vi "Tosca-Plot DI Data.vi"(0 "state in":T2, 5 "Data":cluster{dbl[][], "DI":bool[][]}, 11 "error in (no error)":errorcluster, 12 "Digital":refnum<vi>, 13 "Controls":T1) -> (4 "state out":T2, 15 "error out":errorcluster)   [LabVIEW 2020]
uses:
  Typedefs/Tosca-AI Plot State.ctl
  Typedefs/Tosca-AI Live Controls.ctl
  epl-vi-lib/Utility VIs/Array Manipulation VIs/Array-Dimensions (2D).vi
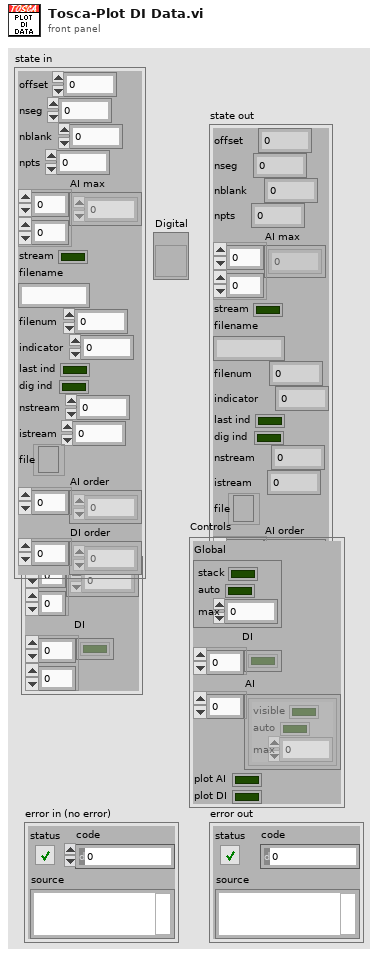
[diagram p1: front panel]
types:
  T1 = typedef "Tosca-AI Live Controls.ctl" = cluster{"Global":cluster{"stack":bool, "auto":bool, "max":dbl}, "DI":bool[], "AI":cluster{"visible":bool, "auto":bool, "max":dbl}[], "plot AI":bool, "plot DI":bool}
  T2 = typedef "Tosca-AI Plot State.ctl" = cluster{"offset":i32, "nseg":i32, "nblank":i32, "npts":i32, "AI max":dbl[][], "stream":bool, "filename":string, "filenum":i32, "indicator":i32, "last ind":bool, "dig ind":bool, "nstream":i32, "istream":i32, "file":refnum<file>, "AI order":i32[], "DI order":i32[]}
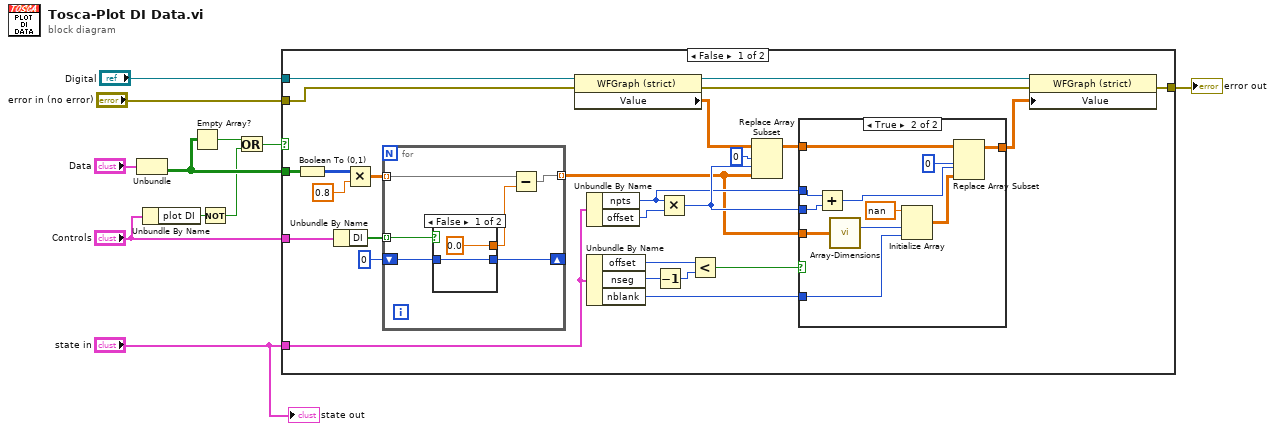
[diagram p0: block diagram]
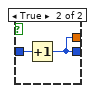
[diagram p2: hidden frame]
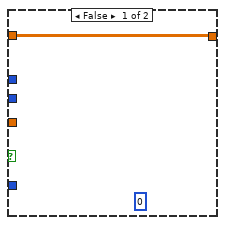
[diagram p3: hidden frame]
diagram:
  n1 = Unbundle("Data") -> ("DI"=w6:bool[][])  [unwired: 1 out]
  n2 = Unbundle By Name("Controls") -> ("plot DI"=w2:bool)
  n3 = Empty Array?(array=w6) -> (empty?=w4:bool)
  n4 = Not(x=w2) -> (.not. x?=w1:bool)
  n5 = Or(x=w4, y=w1) -> (x .or. y?=w3:bool)
  n6 = case shown="False" w3 {
    tunnel: "Digital" -> [w37 _]
    tunnel: "error in (no error)" -> [w36 w60]
    tunnel: "state in" -> [w21 _]
    tunnel: "Controls" -> [w19 _]
    tunnel: [w17 w60] -> w8
    tunnel: w6 -> [w14 _]
    frame False {
      n7 = Boolean To (0,1)(Boolean=w14) -> (0, 1=w12:i16[][])
      n8 = Unbundle By Name(w19) -> ("DI"=w20:bool[])
      n9 = Multiply(x=w12, y=0.8) -> (x*y=w15:dbl[][])
      n10 = for {
        tunnel: w15 -> [w42] mode=indexing
        tunnel: [w43] -> w22 mode=indexing
        tunnel: w20 -> [w38] mode=indexing
        shift-right: [w40] -> _
        shift-left: 0 -> [w41]
        n11 = case shown="False" w38 {
          tunnel: w41 -> [w45 w47]
          tunnel: [w45 w46] -> w40
          tunnel: [0.0 w46] -> w39
          frame False {
          }
          frame True {
            n12 = Increment(x=w47) -> (x+1=w46:i32)
          }
        }
        n13 = Subtract(x=w42, y=w39) -> (x-y=w43:dbl[])
      }
      n14 = property class="WFGraph (strict)"(reference=w37, error in=w36) -> (reference out=w34:refnum<vi>, error out=w33:errorcluster, "Value"=w13:dbl[][])
      n15 = Unbundle By Name(w21) -> ("npts"=w24:i32, "offset"=w32:i32)
      n16 = Unbundle By Name(w21) -> ("offset"=w31:i32, "nseg"=w30:i32, "nblank"=w28:i32)
      n17 = Decrement(x=w30) -> (x-1=w29:i32)
      n18 = Multiply(x=w24, y=w32) -> (x*y=w25:i32)
      n19 = Less?(x=w31, y=w29) -> (x < y?=w26:bool)
      n20 = Replace Array Subset(array=w13, new element=w22, index (row)=0 ("disabled index (row)"), index (col)=w25) -> (w27:dbl[][])
      n21 = case shown="True" w26 {
        tunnel: w22 -> [_ w59]
        tunnel: w28 -> [_ w57]
        tunnel: w27 -> [w48 w55]
        tunnel: w25 -> [_ w52]
        tunnel: w24 -> [_ w51]
        tunnel: [w48 w49] -> w23
        frame False {
          (unwired) 0
        }
        frame True {
          n22 = Add(x=w51, y=w52) -> (x+y=w50:i32)
          n23 = call-poly "Array-Dimensions.vi"("2D Array"=w59) -> ("# rows"=w58:i32)  [unwired: 13 in, 1 out]
          n24 = Initialize Array(nan, w58, w57) -> (w54:dbl[][])
          n25 = Replace Array Subset(array=w55, new element=w54, index (row)=0, index (col)=w50) -> (w49:dbl[][])
        }
      }
      n26 = property class="WFGraph (strict)"(reference=w34, error in=w33, "Value"=w23) -> (error out=w17:errorcluster)  [unwired: 1 out]
    }
    frame True {
    }
  }
  "error out" <- w8
  "state out" <- "state in"
